vi "Subscribe Client.vi"(8 "error in":errorcluster, 10 "Client":string, 11 "Topic in":refnum<class "Topic.lvclass">) -> (0 "error out":errorcluster, 3 "Topic out":refnum<class "Topic.lvclass">)   [LabVIEW 2014, in "Topic.lvclass"]
uses:
  Topic.lvclass
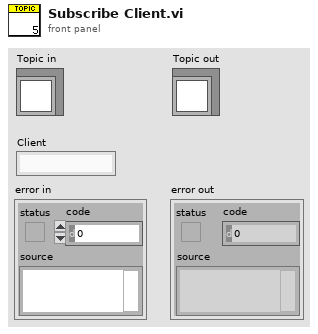
[diagram p1: front panel]
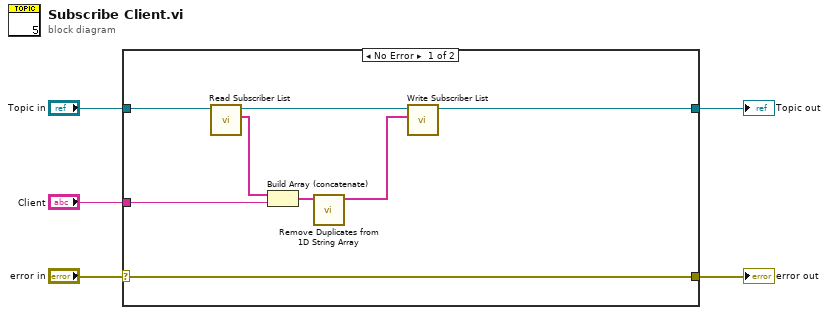
[diagram p0: block diagram]
diagram:
  n1 = case shown="No Error" "error in" {
    selector: "error in" -> [w13 w15]
    tunnel: [w13 w15] -> w4
    tunnel: [w10 w14] -> w2
    tunnel: "Topic in" -> [w12 w14]
    tunnel: "Client" -> [w8 _]
    frame No Error {
      n2 = call-dynamic "Read Subscriber List.vi"("Topic in"=w12) -> ("Subscriber List"=w9:string[], "Topic out"=w11:refnum<class "Topic.lvclass">)  [unwired: 8 in, 1 out]
      n3 = Build Array (concatenate)(w9, w8) -> (w7:string[])
      n4 = call "Remove Duplicates from 1D String Array.vi"("Input Array"=w7) -> ("Output Array"=w6:string[])  [unwired: 10 in]
      n5 = call-dynamic "Write Subscriber List.vi"("Subscriber List"=w6, "Topic in"=w11) -> ("Topic out"=w10:refnum<class "Topic.lvclass">)  [unwired: 8 in, 1 out]
    }
    frame Error {
    }
  }
  "error out" <- w4
  "Topic out" <- w2
